vi "DVSATKdll.vi"(8 "error in (no error)":errorcluster, 11 "Inputs":cluster{"icomp":i32, "t":dbl}) -> (0 "error out":errorcluster, 3 "Outputs":T1)   [LabVIEW 2016]
doc: "subroutine DVSATKdll(icomp, t, D, ierr, herr, herr_length)\n\nCompute pure fluid saturated vapor density with appropriate equation.\n\nINPUTS:\nicomp -- Component i\nt -- Temperature [K]\n\nOUTPUTS:\nD -- Saturated vapor density [mol/L]\nierr --: Error flag: 0 - Successful 1 - T>Tc -2 - D>Dc 501 - No equation available\nherr -- Error string (character*255)\nherr_length -- length of variable herr (default: 255)"
uses:
  REFPROP.DLL
panel:
  # "REFPROP-DVSATKdll.vi"
  # "void  DVSATKdll(int32_t *icomp, double *t, double *D, int32_t *ierr, CStr herr, int32_t *herr_length)"
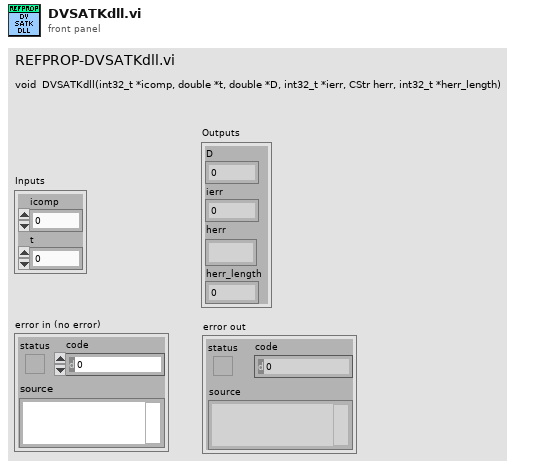
[diagram p1: front panel]
types:
  T1 = cluster{"D":dbl, "ierr":i32, "herr":string, "herr_length":i32}
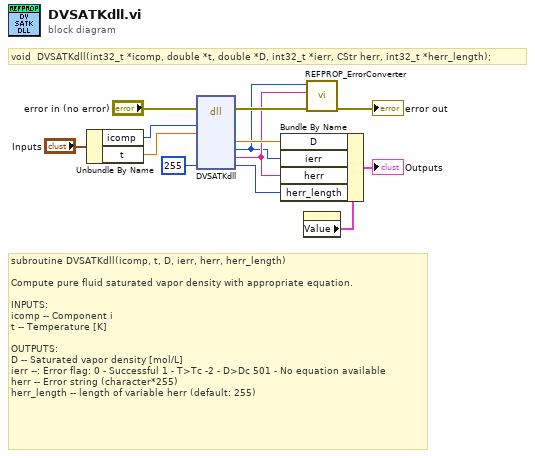
[diagram p0: block diagram]
diagram:
  # "void  DVSATKdll(int32_t *icomp, double *t, double *D, int32_t *ierr, CStr herr, int32_t *herr_length);"
  # "subroutine DVSATKdll(icomp, t, D, ierr, herr, herr_length)\n\nCompute pure fluid saturated vapor density with appropriate equation.\n\nINPUTS:\nicomp -- Component i\nt -- Temperature [K]\n\nOUTPUTS:\nD -- Saturated vapor density [mol/L]\nierr --: Error flag: 0 - Successful 1 - T>Tc -2 - D>Dc 501 - No equation available\nherr -- Error string (character*255)\nherr_length -- length of variable herr (default: 255)"
  n1 = Unbundle By Name("Inputs") -> ("icomp"=w8:i32, "t"=w7:dbl)
  n2 = dll-call lib="S:/009 - Testing/02 - Performance Testing/REFPROP/REFPROP.*" fn="DVSATKdll"(error in="error in (no error)", "icomp"=w8, "t"=w7, "herr_length"=255 ("ln")) -> (error out=w12:errorcluster, "D"=w4:dbl, "ierr"=w1:i32, "herr"=w2:string, "herr_length"=w3:i32)  [unwired: 8 in, 1 out]
  n3 = property on="Outputs" class="Clust (strict)"() -> ("Value"=w6:T1)  [unwired: 2 in, 2 out]
  n4 = Bundle By Name(cluster=w6, "D"=w4, "ierr"=w1, "herr"=w2, "herr_length"=w3) -> (→"Outputs":T1)
  n5 = call "REFPROP_ErrorConverter.vi"("error in (no error)"=w12, "Error Message"=w2, "Error Code"=w1) -> ("error out"=→"error out":errorcluster)  [unwired: 8 in]
